vi "TagMetadataToImage.vi"(8 "error in (no error)":errorcluster, 10 "Image In":T1, 11 "Laser_Oxxius in":refnum<class "Laser_Oxxius.lvclass">) -> (0 "error out":errorcluster, 2 "Image Out":T1, 3 "Laser_Oxxius out":refnum<class "Laser_Oxxius.lvclass">)   [LabVIEW 2020, in "Laser_Oxxius.lvlib" / "Laser_Oxxius.lvclass"]
uses:
  Laser_Oxxius.lvclass
  <vilib>/vision/Image Controls.llb/IMAQ Image.ctl
  Laser_Oxxius.lvclass/Laser_Oxxius.ctl
  Hardware Abstraction Layer/Component/Laser/Laser/Laser.lvclass
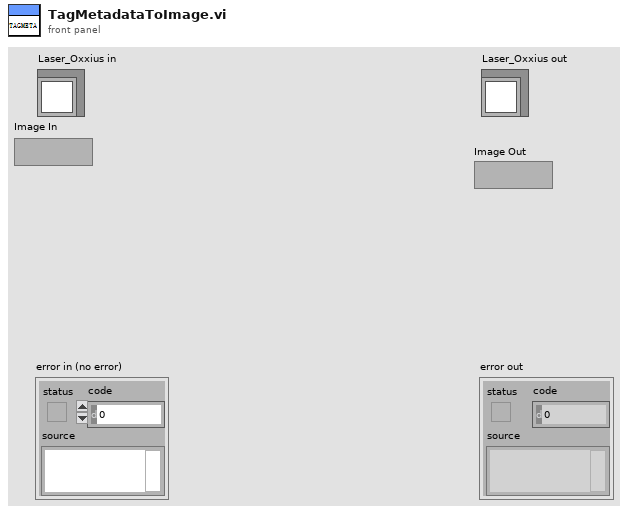
[diagram p1: front panel]
types:
  T1 = typedef "IMAQ Image.ctl" = refnum<image>
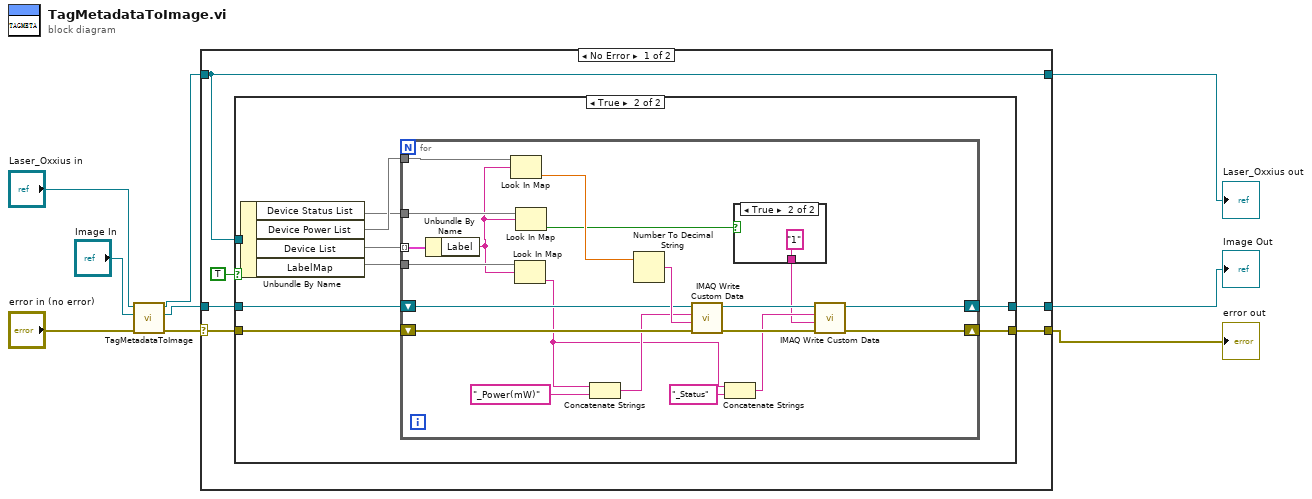
[diagram p0: block diagram]
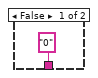
[diagram p3: hidden frame]
diagram:
  n1 = call-parent "TagMetadataToImage.vi"("error in (no error)"="error in (no error)", "Image In"="Image In", "Device in"="Laser_Oxxius in") -> ("error out"=w6:errorcluster, "Image Out"=w5:T1, "Device out"=w4:refnum<class "Laser_Oxxius.lvclass">)  [unwired: 6 in]
  n2 = case shown="No Error" w6 {
    selector: w6 -> [w14 w51]
    tunnel: [w13 w51] -> w1
    tunnel: w5 -> [w12 w50]
    tunnel: [w11 w50] -> w3
    tunnel: [w15 w49] -> w2
    tunnel: w4 -> [w15 w49]
    frame No Error {
      n3 = case shown="True" TRUE {
        tunnel: w15 -> [_ w26]
        tunnel: w14 -> [w16 w25]
        tunnel: [w16 w24] -> w13
        tunnel: w12 -> [w17 w23]
        tunnel: [w17 w22] -> w11
        frame False {
        }
        frame True {
          n4 = Unbundle By Name(w26) -> ("Device Status List"=w19:map{string, bool}, "Device Power List"=w20:map{string, dbl}, "Device List"=w21:map{string, refnum<k24>}, "LabelMap"=w18:map{string, string})
          n5 = for {
            shift-right: [w39] -> w24
            shift-left: w25 -> [w46]
            shift-right: [w37] -> w22
            shift-left: w23 -> [w43]
            tunnel: w21 -> [w42] mode=indexing
            tunnel: w20 -> [w35]
            tunnel: w19 -> [w33]
            tunnel: w18 -> [w29]
            n6 = Unbundle By Name(w42) -> ("Label"=w28:string)
            n7 = Look In Map(map=w35, key=w28) -> (value=w34:dbl)  [unwired: 1 in, 1 out]
            n8 = Look In Map(map=w29, key=w28) -> (value=w27:string)  [unwired: 1 in, 1 out]
            n9 = Look In Map(map=w33, key=w28) -> (value=w32:bool)  [unwired: 1 in, 1 out]
            n10 = Concatenate Strings(w27, "_Power(mW)" ("Key")) -> (w40:string)
            n11 = Number To Decimal String(number=w34) -> (decimal integer string=w44:string)  [unwired: 1 in]
            n12 = call "IMAQ Write Custom Data"("error in (no error)"=w46, "Custom Data In"=w44, "Key"=w40, "Image"=w43) -> ("error out"=w45:errorcluster, "Image Out"=w38:T1)  [unwired: 6 in]
            n13 = Concatenate Strings(w27, "_Status" ("Key")) -> (w31:string)
            n14 = case shown="True" w32 {
              tunnel: ["0" ("Key") "1" ("Key")] -> w30
              frame False {
              }
              frame True {
              }
            }
            n15 = call "IMAQ Write Custom Data"("error in (no error)"=w45, "Custom Data In"=w30, "Key"=w31, "Image"=w38) -> ("error out"=w39:errorcluster, "Image Out"=w37:T1)  [unwired: 6 in]
          }
        }
      }
    }
    frame Error {
    }
  }
  "error out" <- w1
  "Laser_Oxxius out" <- w2
  "Image Out" <- w3
